vi "GFITS_CleanArr2fits.vi"(10 "array":string[][](table)) -> (2 "array out":string[][](table))   [LabVIEW 2016]
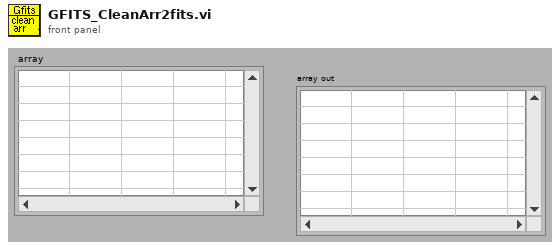
[diagram p1: front panel]
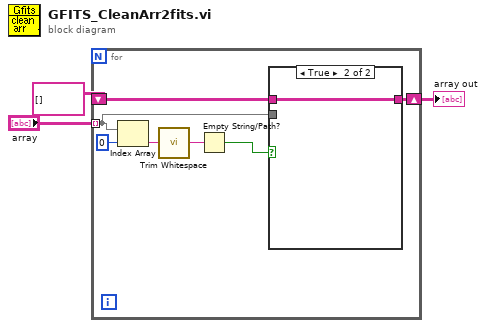
[diagram p0: block diagram]
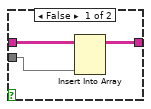
[diagram p2: hidden frame]
diagram:
  n1 = for {
    tunnel: "array" -> [w6] mode=indexing
    shift-right: [w5] -> w1
    shift-left: string[][] [] -> [w4]
    n2 = Index Array(array=w6, index=0) -> (element=w9:string)
    n3 = call <vilib>:"Trim Whitespace.vi"("string"=w9) -> ("trimmed string"=w8:string)  [unwired: 1 in]
    n4 = Empty String/Path?(string/path=w8) -> (empty?=w7:bool)
    n5 = case shown="True" w7 {
      tunnel: w6 -> [w13 _]
      tunnel: [w12 w14] -> w5
      tunnel: w4 -> [w11 w14]
      frame False {
        n6 = Insert Into Array(array=w11, new element=w13) -> (w12:string[][])  [unwired: 2 in]
      }
      frame True {
      }
    }
  }
  "array out" <- w1
